vi "probe_temps.vi"(8 "error in (no error)":errorcluster, 10 "locations":string[](array[string]), 11 "TempProbeSet in":refnum<class "TempProbeSet.lvclass">) -> (0 "error out":errorcluster, 2 "temps":dbl[](array[numeric]), 3 "TempProbeSet out":refnum<class "TempProbeSet.lvclass">)   [LabVIEW 2010, in "TempProbeSet.lvclass"]
doc: "This VI takes in a TempProbeSet object and an array of location strings and spits out the corresponding array of temperature values. This VI first looks to see if the TempProbeSet (which is initialized off of the temperature probe calibration file) has at probe with the location string passed as an entry within the \"location\" strings input. If it finds a match, then it procedes in calling the process_probe_resistance_array method on the matching TempProbe objects. If not, it passes an error out of this VI along with a -/inf numeric for the corresponding temperature value."
uses:
  TempProbeSet.lvclass
  TempProbe.lvclass
  accessors/read_probes.vi
  accessors/read_probe_keys.vi
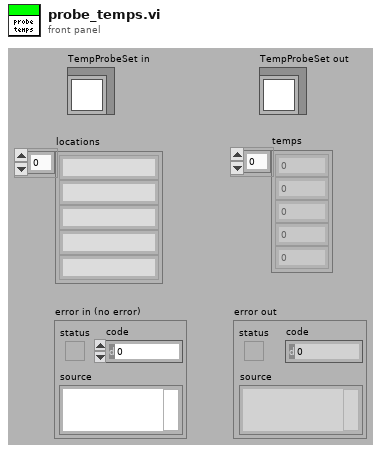
[diagram p1: front panel]
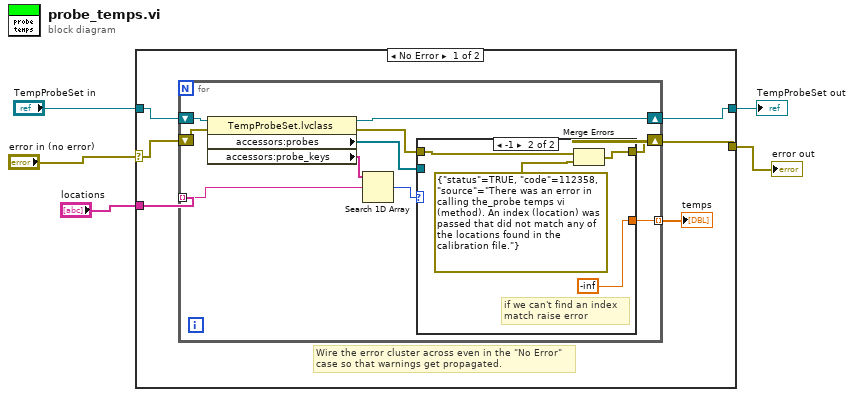
[diagram p0: block diagram]
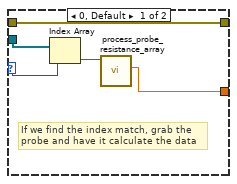
[diagram p2: hidden frame]
diagram:
  n1 = case shown="No Error" "error in (no error)" {
    selector: "error in (no error)" -> [w8 w32]
    tunnel: [w7 w32] -> w4
    tunnel: [w9 w31] -> w2
    tunnel: "TempProbeSet in" -> [w10 w31]
    tunnel: "locations" -> [w11 _]
    frame No Error {
      # "Wire the error cluster across even in the \"No Error\"\ncase so that warnings get propagated."
      n2 = for {
        tunnel: w11 -> [w19] mode=indexing
        shift-right: [w18] -> w9
        shift-left: w10 -> [w21]
        shift-right: [w13] -> w7
        shift-left: w8 -> [w20]
        tunnel: [w12] -> w6 mode=indexing
        n3 = property class="TempProbeSet.lvclass"(reference=w21, error in=w20) -> (reference out=w18:refnum<class "TempProbeSet.lvclass">, error out=w14:errorcluster, "accessors:probes"=w16:refnum<class "TempProbe.lvclass">[], "accessors:probe_keys"=w17:string[])
        n4 = Search 1D Array(1D array=w17, element=w19) -> (index of element=w15:i32)  [unwired: 1 in]
        n5 = case shown="-1" w15 {
          selector: w15 -> [w24 _]
          tunnel: w16 -> [w26 _]
          tunnel: w14 -> [w23 w30]
          tunnel: [w23 w29] -> w13
          tunnel: [w22 -inf] -> w12
          frame 0, Default {
            # "If we find the index match, grab the\nprobe and have it calculate the data"
            n6 = Index Array(array=w26, index=w24) -> (element=w25:refnum<class "TempProbe.lvclass">)
            n7 = call "process_probe_resistance_array.vi"("TempProbe in"=w25) -> ("temperature"=w22:dbl)  [unwired: 6 in, 4 out]
          }
          frame -1 {
            # "if we can't find an index\nmatch raise error"
            n8 = Merge Errors(w30, errorcluster {"status"=TRUE, "code"=112358, "source"="There was an error in calling the_probe temps vi (method). An index (location) was passed that did not match any of the locations found in the calibration file."} ("bad location index error")) -> (w29:errorcluster)
          }
        }
      }
      "temps" <- w6
    }
    frame Error {
    }
  }
  "error out" <- w4
  "TempProbeSet out" <- w2
